vi "Lvi Read U16Data1D.vi"(7 "OnlyReadAvailable":bool, 8 "error in (no error)":errorcluster, 9 "timeout":dbl, 10 "TaskRef":i32, 11 "DataBufSize":u32) -> (0 "error out":errorcluster, 1 "DataBuf":u16[](array[numeric]), 2 "TaskRef out":i32, 3 "DataBufSize out":u32, 5 "function return":i32)   [LabVIEW 2022 SP3, in "DtLvLink.lvlib"]
doc: "Calls directly into the entry points of the DLL of the Data Acq SDK to return a data point from the specified task as an unsigned 16-bit integer. \n\n \n\n\n\n\n\nLvErrorCode LviReadI16Data1D(unsigned int *DataBufSize, short *DataBuf, LvTaskRef * TaskRef,\n double timeout, bool OnlyReadAvailable);"
uses:
  DtLvLink.lvlib
  <userlib>/LV-Link3/DtLvLink_64.dll
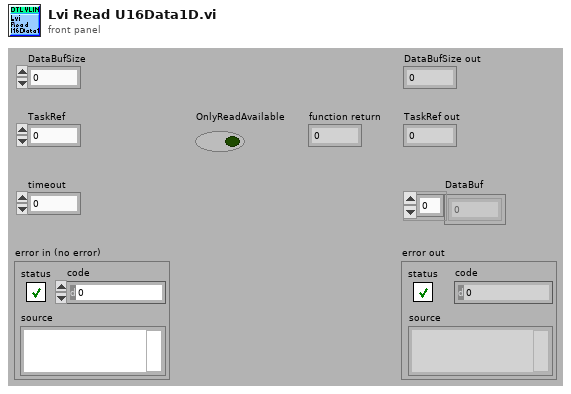
[diagram p1: front panel]
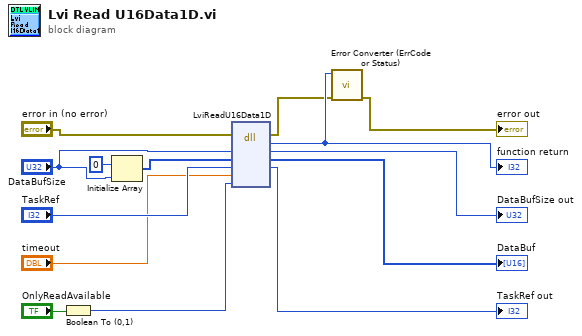
[diagram p0: block diagram]
diagram:
  n1 = Boolean To (0,1)(Boolean="OnlyReadAvailable") -> (0, 1=w4:i16)
  n2 = Initialize Array(u16 0 ("element"), "DataBufSize") -> (w11:u16[])
  n3 = dll-call lib="C:/Program Files/National Instruments/LabVIEW 2022/user.lib/LV-Link3/DtLvLink_64.*" fn="LviReadU16Data1D"(error in="error in (no error)", "DataBufSize"="DataBufSize", "DataBuf"=w11, "TaskRef"="TaskRef", "timeout"="timeout", "OnlyReadAvailable"=w4) -> (error out=w2:errorcluster, "return type"=w14:i32, "DataBufSize"=→"DataBufSize out":u32, "DataBuf"=→"DataBuf":u16[], "TaskRef"=→"TaskRef out":i32)  [unwired: 4 in, 1 out]
  "function return" <- w14
  n4 = call "Error Converter (ErrCode or Status).vi"("error in (no error)"=w2, "error code"=w14) -> ("error out"=→"error out":errorcluster)  [unwired: 9 in]
